vi "Wait For Packet.vi"(7 "Timeout (100 ms)":u32=100, 8 "Error In":errorcluster, 11 "LINX Device Config":T1) -> (0 "Error Out":errorcluster, 2 "Packet":u8[](array[numeric]), 3 "LINX Device Config":T1)   [LabVIEW 2011, in "LVH-LINX.lvlib" / "Device.lvlib"]
doc: "Wait until a LINX return packet is received or a timout occurs. If a valid packet is recieved this VI will return that packet otherwise this VI returns and empty packet and generates an error."
uses:
  Device.lvlib
  Type Defs/LINX Device Config.ctl
  Type Defs/Interface.ctl
  Type Defs/TCP Config.ctl
  Type Defs/Device Family.ctl
  Type Defs/Error Type.ctl
  LVH-LINX.lvlib
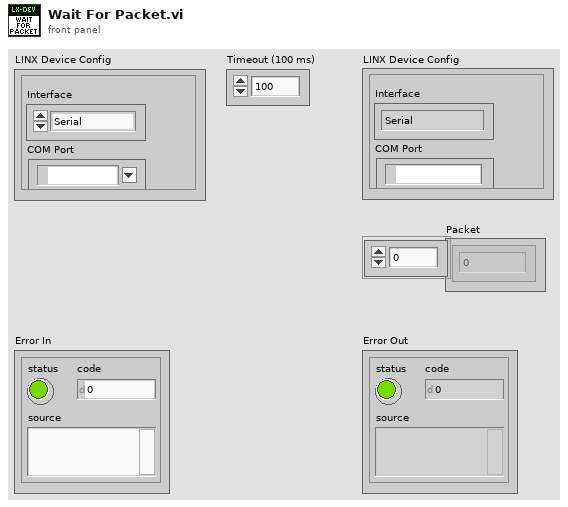
[diagram p1: front panel]
types:
  T1 = typedef "LVH-LINX.lvlib/Device.lvlib/LINX Device Config.ctl" = cluster{"Interface":T2, "COM Port":refnum<visa-resource-name>, "TCP Configuration":T3, "Device Family":T4, "Device ID":u8, "Device Name":string, "TCP Ref":refnum<k5>}
  T2 = typedef "LVH-LINX.lvlib/Interface.ctl" = enum16{"Serial", "TCP"}
  T3 = typedef "LVH-LINX.lvlib/Device.lvlib/TCP Config.ctl" = cluster{"IP Address":string, "Port":u16}
  T4 = typedef "LVH-LINX.lvlib/Device Family.ctl" = enum8{"National Instruments", "Digilent", "Arduino"}
  T5 = typedef "LVH-LINX.lvlib/Error Type.ctl" = enum16{"Unknown", "Timeout", "Corrupt Return Packet", "Unable To Connect", "Command Not Supported", "Channel DNE"}
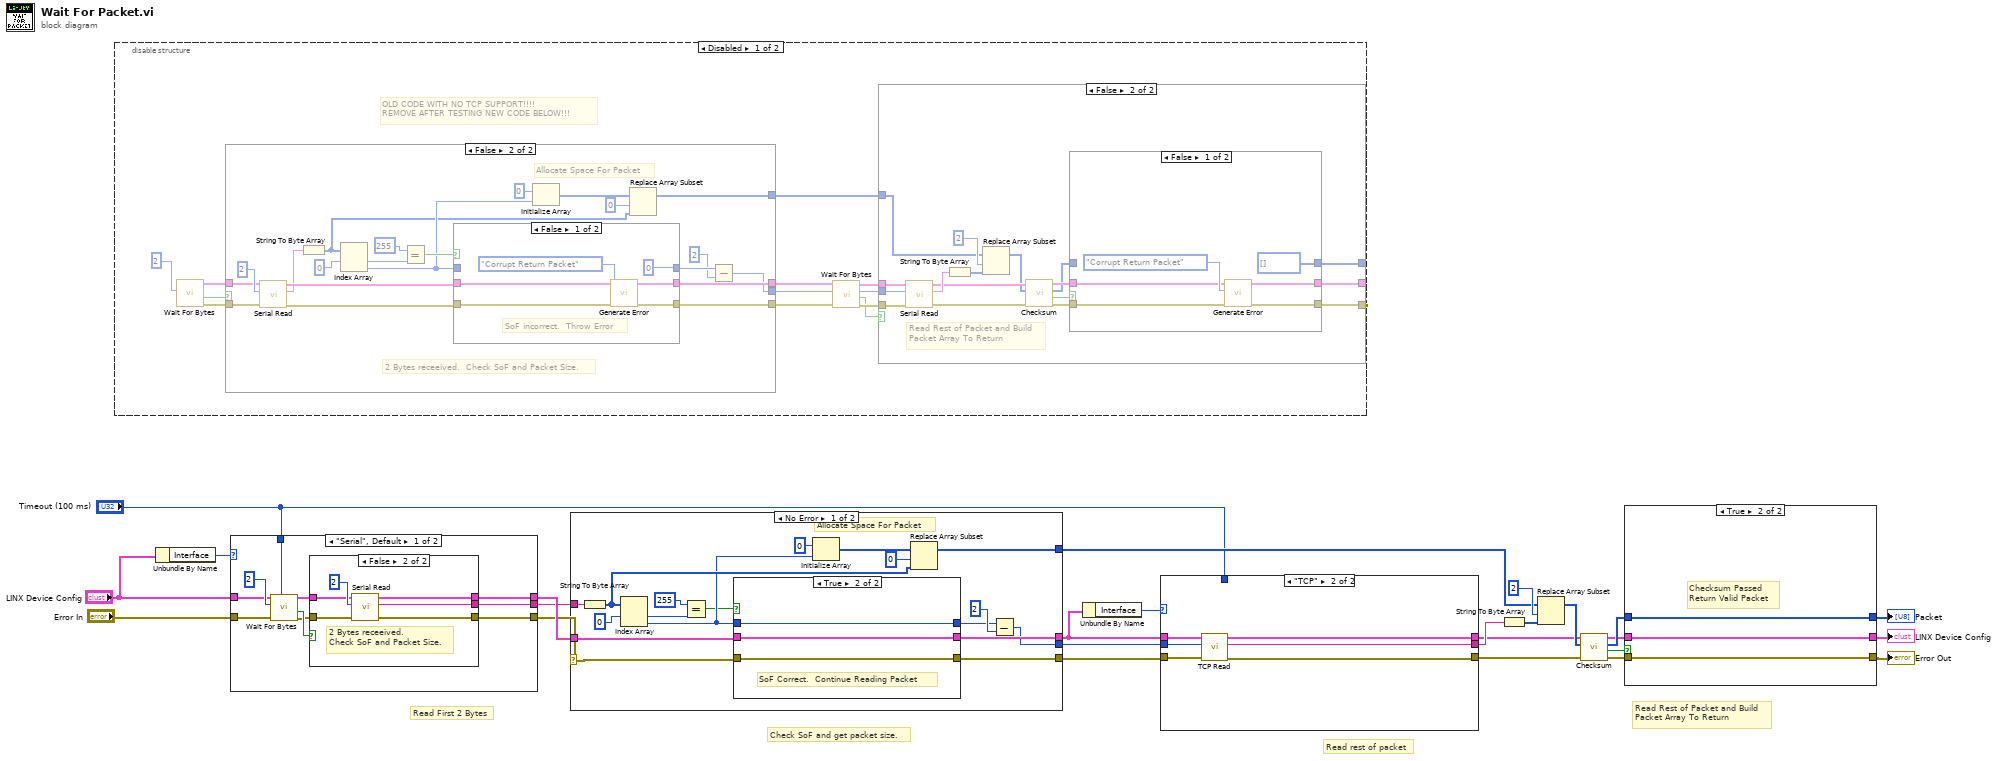
[diagram p0: block diagram]
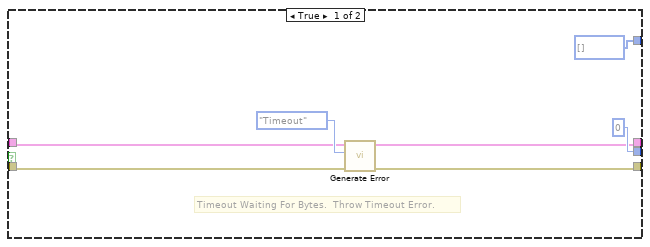
[diagram p2: hidden frame]
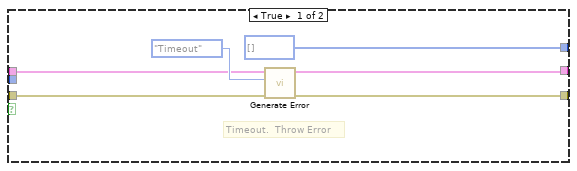
[diagram p4: hidden frame]
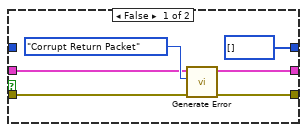
[diagram p7: hidden frame]
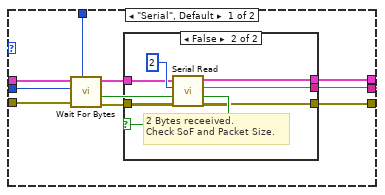
[diagram p8: hidden frame]
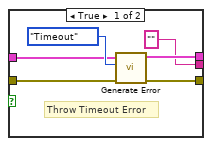
[diagram p9: hidden frame]
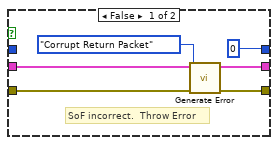
[diagram p10: hidden frame]
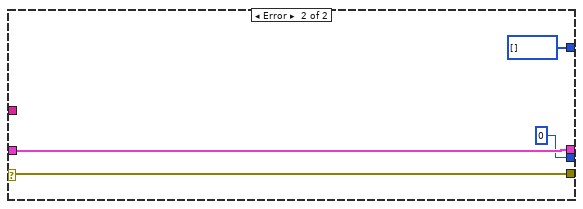
[diagram p11: hidden frame]
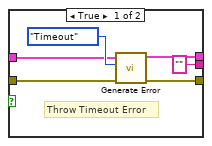
[diagram p12: hidden frame]
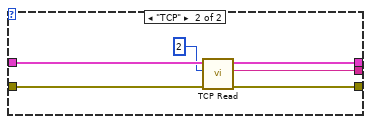
[diagram p13: hidden frame]
diagram:
  # "Read Rest of Packet and Build\nPacket Array To Return"
  # "Read rest of packet"
  # "Check SoF and get packet size."
  # "Read First 2 Bytes"
  n1 = disable-structure shown="Disabled" {
    frame Disabled {
      # "OLD CODE WITH NO TCP SUPPORT!!!!\nREMOVE AFTER TESTING NEW CODE BELOW!!!"
      n2 = call "Wait For Bytes.vi"("Num Bytes"=u32 2) -> ("Error Out"=w37:errorcluster, "Timeout"=w29:bool, "LINX Device Config"=w36:T1)  [unwired: 7 in, 1 out]
      n3 = case shown="False" w29 {
        tunnel: w37 -> [w42 w53]
        tunnel: w36 -> [w38 w51]
        tunnel: [u8 0 w45] -> w34
        tunnel: [w41 w61] -> w32
        tunnel: [w39 w54] -> w33
        tunnel: [u8[] [] w55] -> w26
        frame True {
          # "Timeout Waiting For Bytes.  Throw Timeout Error."
          n4 = call "Generate Error.vi"("Error In"=w42, "Error Type"=Error_Type."Timeout", "LINX Device Config"=w38) -> ("Error Out"=w41:errorcluster, "LINX Device Config"=w39:T1)  [unwired: 7 in]
        }
        frame False {
          # "Allocate Space For Packet"
          # "2 Bytes receeived.  Check SoF and Packet Size."
          n5 = call "Serial Read.vi"("Error In"=w53, "Bytes To Read"=u32 2 ("byte count"), "LINX Device Config"=w51) -> ("Error Out"=w49:errorcluster, "Data"=w48:string, "LINX Device Config"=w50:T1)  [unwired: 6 in]
          n6 = String To Byte Array(string=w48) -> (unsigned byte array=w56:u8[])
          n7 = Index Array(array=w56, index #1=0 ("index")) -> (element #1=w64:u8, element #2=w60:u8)  [unwired: 1 in]
          n8 = Equal?(x=u8 255, y=w64) -> (x = y?=w62:bool)
          n9 = case shown="False" w62 {
            tunnel: w60 -> [_ w72]
            tunnel: w49 -> [w71 w74]
            tunnel: [w70 w74] -> w61
            tunnel: [w67 w73] -> w54
            tunnel: w50 -> [w68 w73]
            tunnel: [u8 0 w72] -> w47
            frame False {
              # "SoF incorrect.  Throw Error"
              n10 = call "Generate Error.vi"("Error In"=w71, "Error Type"=Error_Type."Corrupt Return Packet", "LINX Device Config"=w68) -> ("Error Out"=w70:errorcluster, "LINX Device Config"=w67:T1)  [unwired: 7 in]
            }
            frame True {
              # "SoF Correct.  Continue Reading Packet"
            }
          }
          n11 = Initialize Array(u8 0 ("element"), w60) -> (w58:u8[])
          n12 = Replace Array Subset(array=w58, new element=w56, index=0) -> (w55:u8[])
          n13 = Subtract(x=w47, y=u8 2) -> (x-y=w45:u8)
        }
      }
      n14 = call "Wait For Bytes.vi"("Error In"=w32, "Num Bytes"=w34, "LINX Device Config"=w33) -> ("Error Out"=w31:errorcluster, "Timeout"=w27:bool, "Num Bytes"=w28:u32, "LINX Device Config"=w30:T1)  [unwired: 5 in]
      n15 = case shown="False" w27 {
        tunnel: w31 -> [w79 w92]
        tunnel: w30 -> [w76 w93]
        tunnel: w28 -> [_ w91]
        tunnel: [w78 w95] -> _
        tunnel: [w75 w94] -> _
        tunnel: w26 -> [_ w89]
        tunnel: [u8[] [] ("unsigned byte array") w81] -> _
        frame True {
          # "Timeout.  Throw Error"
          n16 = call "Generate Error.vi"("Error In"=w79, "Error Type"=Error_Type."Timeout", "LINX Device Config"=w76) -> ("Error Out"=w78:errorcluster, "LINX Device Config"=w75:T1)  [unwired: 7 in]
        }
        frame False {
          # "Read Rest of Packet and Build\nPacket Array To Return"
          n17 = call "Serial Read.vi"("Error In"=w92, "Bytes To Read"=w91, "LINX Device Config"=w93) -> ("Error Out"=w88:errorcluster, "Data"=w90:string, "LINX Device Config"=w87:T1)  [unwired: 6 in]
          n18 = String To Byte Array(string=w90) -> (unsigned byte array=w96:u8[])
          n19 = Replace Array Subset(array=w89, new element=w96, index=2) -> (w86:u8[])
          n20 = call "Checksum.vi"("Error In"=w88, "Packet"=w86, "LINX Device Config"=w87) -> ("Error Out"=w84:errorcluster, "Checksum Pass?"=w83:bool, "Packet"=w82:u8[], "LINX Device Config"=w85:T1)  [unwired: 5 in]
          n21 = case shown="False" w83 {
            tunnel: [w103 w106] -> w95
            tunnel: w84 -> [w102 w106]
            tunnel: [w99 w105] -> w94
            tunnel: w85 -> [w100 w105]
            tunnel: w82 -> [_ w104]
            tunnel: [u8[] [] w104] -> w81
            frame False {
              n22 = call "Generate Error.vi"("Error In"=w102, "Error Type"=Error_Type."Corrupt Return Packet", "LINX Device Config"=w100) -> ("Error Out"=w103:errorcluster, "LINX Device Config"=w99:T1)  [unwired: 7 in]
            }
            frame True {
              # "Checksum Passed\nReturn Valid Packet"
            }
          }
        }
      }
    }
    frame Enabled {
    }
  }
  n23 = Unbundle By Name("LINX Device Config") -> ("Interface"=w25:T2)
  n24 = case shown="\"Serial\", Default" w25 {
    tunnel: "Error In" -> [w115 w133]
    tunnel: "LINX Device Config" -> [w114 w134]
    tunnel: [w110 w132] -> w22
    tunnel: [w109 w131] -> w21
    tunnel: [w108 w129] -> w20
    tunnel: "Timeout (100 ms)" -> [w107 _]
    frame "Serial", Default {
      n25 = call "Wait For Bytes.vi"("Timeout (100 ms)"=w107, "Error In"=w115, "Num Bytes"=u32 2, "LINX Device Config"=w114) -> ("Error Out"=w111:errorcluster, "Timeout"=w113:bool, "LINX Device Config"=w112:T1)  [unwired: 4 in, 1 out]
      n26 = case shown="False" w113 {
        tunnel: w112 -> [w121 w127]
        tunnel: w111 -> [w120 w126]
        tunnel: [w119 w125] -> w110
        tunnel: [w118 w124] -> w109
        tunnel: ["" ("Data") w123] -> w108
        frame True {
          # "Throw Timeout Error"
          n27 = call "Generate Error.vi"("Error In"=w120, "Error Type"=Error_Type."Timeout", "LINX Device Config"=w121) -> ("Error Out"=w118:errorcluster, "LINX Device Config"=w119:T1)  [unwired: 7 in]
        }
        frame False {
          # "2 Bytes receeived.  \nCheck SoF and Packet Size."
          n28 = call "Serial Read.vi"("Error In"=w126, "Bytes To Read"=u32 2 ("byte count"), "LINX Device Config"=w127) -> ("Error Out"=w124:errorcluster, "Data"=w123:string, "LINX Device Config"=w125:T1)  [unwired: 6 in]
        }
      }
    }
    frame "TCP" {
      n29 = call "TCP Read.vi"("Error In"=w133, "Bytes To Read"=u32 2 ("Num Bytes"), "LINX Device Config"=w134) -> ("Error Out"=w131:errorcluster, "Data"=w129:string, "LINX Device Config"=w132:T1)  [unwired: 6 in]
    }
  }
  n30 = case shown="No Error" w21 {
    selector: w21 -> [w140 w164]
    tunnel: w22 -> [w141 w165]
    tunnel: w20 -> [w139 _]
    tunnel: [w138 u8[] []] -> w6
    tunnel: [w137 w165] -> w19
    tunnel: [w136 w164] -> w17
    tunnel: [w135 u8 0] -> w1
    frame No Error {
      # "Allocate Space For Packet"
      n31 = String To Byte Array(string=w139) -> (unsigned byte array=w150:u8[])
      n32 = Index Array(array=w150, index #1=0 ("index")) -> (element #1=w143:u8, element #2=w146:u8)  [unwired: 1 in]
      n33 = Equal?(x=u8 255, y=w143) -> (x = y?=w145:bool)
      n34 = case shown="True" w145 {
        tunnel: w146 -> [_ w159]
        tunnel: w140 -> [w158 w161]
        tunnel: [w157 w161] -> w136
        tunnel: [w154 w160] -> w137
        tunnel: w141 -> [w155 w160]
        tunnel: [u8 0 w159] -> w151
        frame False {
          # "SoF incorrect.  Throw Error"
          n35 = call "Generate Error.vi"("Error In"=w158, "Error Type"=Error_Type."Corrupt Return Packet", "LINX Device Config"=w155) -> ("Error Out"=w157:errorcluster, "LINX Device Config"=w154:T1)  [unwired: 7 in]
        }
        frame True {
          # "SoF Correct.  Continue Reading Packet"
        }
      }
      n36 = Initialize Array(u8 0 ("element"), w146) -> (w148:u8[])
      n37 = Replace Array Subset(array=w148, new element=w150, index=0) -> (w138:u8[])
      n38 = Subtract(x=w151, y=u8 2) -> (x-y=w135:u8)
    }
    frame Error {
    }
  }
  n39 = Unbundle By Name(w19) -> ("Interface"=w18:T2)
  n40 = case shown="\"TCP\"" w18 {
    tunnel: w17 -> [w175 w192]
    tunnel: w19 -> [w174 w193]
    tunnel: [w170 w190] -> w7
    tunnel: [w169 w191] -> w9
    tunnel: [w168 w189] -> w8
    tunnel: "Timeout (100 ms)" -> [w167 _]
    tunnel: w1 -> [w166 w188]
    frame "Serial", Default {
      n41 = call "Wait For Bytes.vi"("Timeout (100 ms)"=w167, "Error In"=w175, "Num Bytes"=w166, "LINX Device Config"=w174) -> ("Error Out"=w171:errorcluster, "Timeout"=w173:bool, "LINX Device Config"=w172:T1)  [unwired: 4 in, 1 out]
      n42 = case shown="False" w173 {
        tunnel: w172 -> [w180 w186]
        tunnel: w171 -> [w179 w185]
        tunnel: [w178 w184] -> w170
        tunnel: [w177 w183] -> w169
        tunnel: ["" ("Data") w182] -> w168
        frame True {
          # "Throw Timeout Error"
          n43 = call "Generate Error.vi"("Error In"=w179, "Error Type"=Error_Type."Timeout", "LINX Device Config"=w180) -> ("Error Out"=w177:errorcluster, "LINX Device Config"=w178:T1)  [unwired: 7 in]
        }
        frame False {
          # "2 Bytes receeived.  \nCheck SoF and Packet Size."
          n44 = call "Serial Read.vi"("Error In"=w185, "Bytes To Read"=u32 2 ("byte count"), "LINX Device Config"=w186) -> ("Error Out"=w183:errorcluster, "Data"=w182:string, "LINX Device Config"=w184:T1)  [unwired: 6 in]
        }
      }
    }
    frame "TCP" {
      n45 = call "TCP Read.vi"("Error In"=w192, "Bytes To Read"=w188, "LINX Device Config"=w193) -> ("Error Out"=w191:errorcluster, "Data"=w189:string, "LINX Device Config"=w190:T1)  [unwired: 6 in]
    }
  }
  n46 = String To Byte Array(string=w8) -> (unsigned byte array=w11:u8[])
  n47 = Replace Array Subset(array=w6, new element=w11, index=2) -> (w12:u8[])
  n48 = call "Checksum.vi"("Error In"=w9, "Packet"=w12, "LINX Device Config"=w7) -> ("Error Out"=w14:errorcluster, "Checksum Pass?"=w15:bool, "Packet"=w16:u8[], "LINX Device Config"=w13:T1)  [unwired: 5 in]
  n49 = case shown="True" w15 {
    tunnel: [w199 w202] -> w5
    tunnel: w14 -> [w198 w202]
    tunnel: [w195 w201] -> w4
    tunnel: w13 -> [w196 w201]
    tunnel: w16 -> [_ w200]
    tunnel: [u8[] [] w200] -> w3
    frame False {
      n50 = call "Generate Error.vi"("Error In"=w198, "Error Type"=Error_Type."Corrupt Return Packet", "LINX Device Config"=w196) -> ("Error Out"=w199:errorcluster, "LINX Device Config"=w195:T1)  [unwired: 7 in]
    }
    frame True {
      # "Checksum Passed\nReturn Valid Packet"
    }
  }
  "Error Out" <- w5
  "Packet" <- w3
  "LINX Device Config" <- w4
